vi "feedforward_estimation.vi"(2 "Parameters":T1={"Stimulus"={"Type"=enum."Off", "Phase"=0.0, "Amplitude"=[], "Injection point"=enum."Total pose", "Closed loop"=FALSE, "Offset"=[], "Tip -> world"=FALSE, "Frequency"=0.0, "Length"=0.0}, "Goal Filter A"={"Speedup max"=0.0, "Speedup thresh"=0.0, "Speedup nonlin"=0.0, "Filters"=[]}, "Mode controls"={"Hold"=FALSE, "Cancellation"=FALSE, "Goal filter"=FALSE, "Trigger"=FALSE}, "Manipulator type"=enum."Current piezo", "Manipulator calibration"={"Tool offsets"=[], "Tip light calibration"=[], "Handle light calibration"=[], "Base pivots"=[], "Output pivots"=[], "Length center"=0.0, "Workspace height"=[], "Workspace diameter"=[0.0, 0.0, 36200.0], "Linearization"=[[0.0, 0.0, 36200.0]], "Stack travel"=400.0, "Saturation pos"=375.0, "Inverse filters"=[]}, "Network"={"Remote Host"="", "Send Status"=FALSE, "Send Port"=0, "Recv Commands"=FALSE, "Recv Port"=0}, "Goal Filter B"={"Speedup max"=0.0, "Speedup thresh"=0.0, "Speedup nonlin"=0.0, "Filters"=[]}, "Cancellation"={"KP"={"XY"=0.0, "Rxy"=0.0, "Z"=0.0, "Rz"=0.0}, "KI"=0.0, "KD"={"XY"=0.0, "Rxy"=0.0, "Z"=0.0, "Rz"=0.0}, "Max vel"=0.0, "Max acc"=0.0, "Int error limit"=0.0, "RCM gain"=0.0, "Bypass"=FALSE, "Degraded gain"=0.0}, "Transition time"=0.0, "Estimation"={"Link"={"Measure noise"=[], "Process noise"=[], "Alt process noise"=[], "Alt turnoff cycles"=20, "Innovation limit"=[], "Residue threshold"=0.0, "Enable"=FALSE}, "Handle"={"Measure noise"=[], "Process noise"=[], "State limits"=[], "Innovation limit"=[], "Prediction Lookahead"=0.0, "Enable"=FALSE}}} {"Transition time" format="%_3f"; "Cancellation"."Degraded gain" min=0 max=1 step=0.1 format="%#_3p"; "Cancellation"."RCM gain" min=0 max=1 step=0.1 format="%#_3p"; "Cancellation"."KD"."Rz" min=0 max=1 step=0.1 format="%#_3p"; "Cancellation"."KD"."Rxy" min=0 max=1 step=0.1 format="%#_3p"; "Cancellation"."KD"."Z" min=0 max=1 step=0.1 format="%#_3p"; "Cancellation"."KD"."XY" min=0 max=1 step=0.1 format="%#_3p"; "Cancellation"."KI" min=0 max=1 step=0.01 format="%#_3p"; "Cancellation"."KP"."Rz" min=0 max=1 step=0.1 format="%#_3p"; "Cancellation"."KP"."Rxy" min=0 max=1 step=0.1 format="%#_3p"; "Cancellation"."KP"."Z" min=0 max=1 step=0.1 format="%#_3p"; "Cancellation"."KP"."XY" min=0 max=1 step=0.1 format="%#_3p"; "Cancellation"."Max acc" format="%#_3p"; "Goal Filter B"."Filters"."V limit range" format="%_3p"; "Goal Filter B"."Filters"."V limit" format="%_3p"; "Goal Filter B"."Filters"."Upper Q" format="%_3f"; "Goal Filter B"."Filters"."Upper Fc" format="%_3p"; "Goal Filter B"."Filters"."Lower Q" format="%_3f"; "Goal Filter B"."Filters"."Scale factor" format="%_3f"; "Goal Filter B"."Filters"."Lower Fc" format="%_3p"; "Goal Filter B"."Speedup nonlin" format="%_3p"; "Goal Filter B"."Speedup thresh" format="%_3p"; "Goal Filter B"."Speedup max" format="%_3p"; "Manipulator calibration"."Saturation pos" format="%#.1f"; "Manipulator calibration"."Stack travel" format="%#.1f"; "Manipulator calibration"."Output pivots" format="%#_6f"; "Manipulator calibration"."Base pivots" format="%#_6f"; "Manipulator calibration"."Handle light calibration" format="%#.1f"; "Manipulator calibration"."Tip light calibration" format="%#.1f"; "Goal Filter A"."Filters"."V limit range" format="%_3p"; "Goal Filter A"."Filters"."V limit" format="%_3p"; "Goal Filter A"."Filters"."Upper Q" format="%_3f"; "Goal Filter A"."Filters"."Upper Fc" format="%_3p"; "Goal Filter A"."Filters"."Lower Q" format="%_3f"; "Goal Filter A"."Filters"."Scale factor" format="%_3f"; "Goal Filter A"."Filters"."Lower Fc" format="%_3p"; "Goal Filter A"."Speedup nonlin" format="%_3p"; "Goal Filter A"."Speedup thresh" format="%_3p"; "Goal Filter A"."Speedup max" format="%_3p"; "Stimulus"."Length" min=0.0 max=100.0 step=100.0 format="%#_4p"; "Stimulus"."Frequency" min=0.0 step=100.0 format="%#_4g"; "Stimulus"."Offset" format="%#_3p"; "Stimulus"."Amplitude" format="%#_3p"; "Stimulus"."Phase" min=-180.0 max=360.0 step=100.0 format="%#.2f"}, 3 "Handle Velocity":dbl[](array[numeric]), 4 "Handle Acceleration":dbl[](array[numeric])) -> (5 "Prediction":dbl[](array[numeric]))   [LabVIEW 2013]
uses:
  <vilib>/Analysis/NI_AALBase.lvlib
  <vilib>/Analysis/baseanly.llb/A x Vector.vi
  testing/injection_point.ctl
  testing/stimulus.ctl
  testing/mode_conrols.ctl
  asap/labview/testing/probe_calibration.ctl
  testing/manipulator_cal.ctl
  host/network_params.ctl
  testing/Micron params.ctl
  goal_loop_parms.ctl
  cancellation/decoupled_gain.ctl
  cancellation/sq_control_params.ctl
  cancellation/estimation_controls.ctl
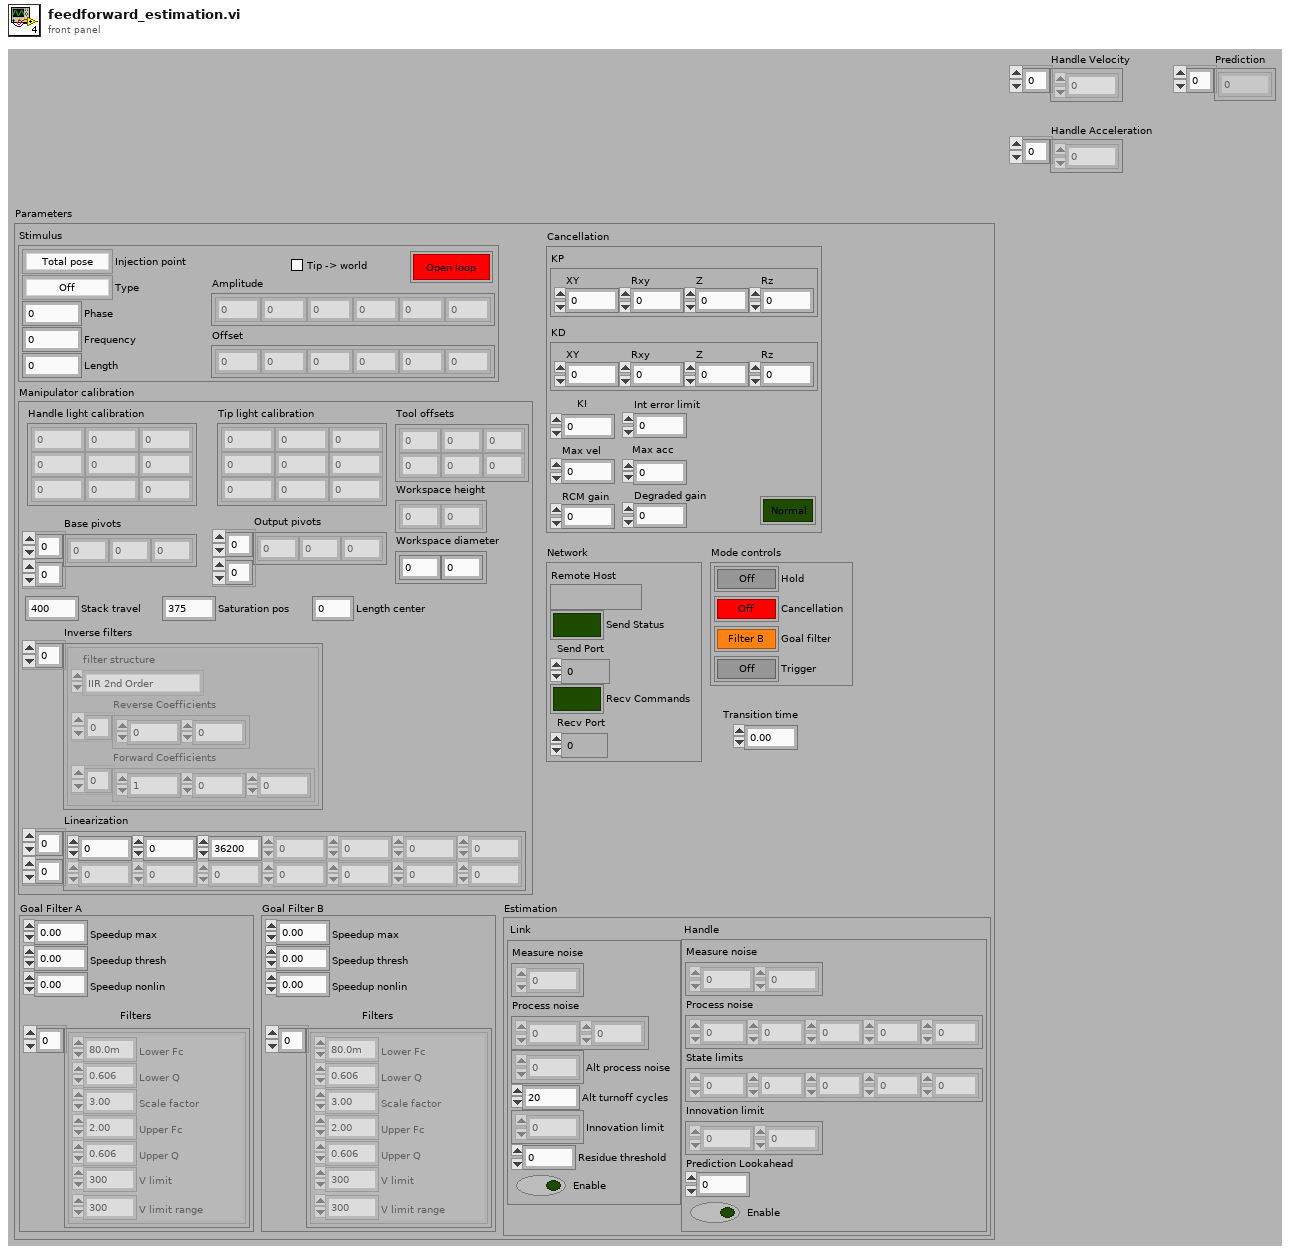
[diagram p1: front panel]
types:
  T1 = typedef "Micron params.ctl" = cluster{"Stimulus":T2, "Goal Filter A":T4, "Mode controls":T5, "Manipulator type":enum16{"Current piezo", "Voltage piezo"}, "Manipulator calibration":T6, "Network":T8, "Goal Filter B":T4, "Cancellation":T9, "Transition time":sgl, "Estimation":T11}
  T2 = typedef "stimulus.ctl" = cluster{"Type":enum16{"Off", "Step", "Sine", "Triangle", "Arbitrary"}, "Phase":dbl, "Amplitude":sgl[], "Injection point":T3, "Closed loop":bool, "Offset":sgl[], "Tip -> world":bool, "Frequency":dbl, "Length":dbl}
  T3 = typedef "injection_point.ctl" = enum16{"Total pose", "V limiter", "Goal ", "Link position", "KF link position", "Inverse kin", "Link goal", "Link error", "Controller", "Output", "Drive", "Light"}
  T4 = typedef "goal_loop_parms.ctl" = cluster{"Speedup max":sgl, "Speedup thresh":sgl, "Speedup nonlin":sgl, "Filters":cluster{"Lower Fc":sgl, "Lower Q":sgl, "Scale factor":sgl, "Upper Fc":sgl, "Upper Q":sgl, "V limit":sgl, "V limit range":sgl}[]}
  T5 = typedef "mode_conrols.ctl" = cluster{"Hold":bool, "Cancellation":bool, "Goal filter":bool, "Trigger":bool}
  T6 = typedef "manipulator_cal.ctl" = cluster{"Tool offsets":sgl[][], "Tip light calibration":T7, "Handle light calibration":T7, "Base pivots":sgl[][], "Output pivots":sgl[][], "Length center":sgl, "Workspace height":sgl[], "Workspace diameter":sgl[], "Linearization":sgl[][], "Stack travel":sgl, "Saturation pos":sgl, "Inverse filters":cluster{"filter structure":enum32{"IIR 2nd Order", "IIR 4th Order"}, "Reverse Coefficients":dbl[], "Forward Coefficients":dbl[]}[]}
  T7 = typedef "probe_calibration.ctl" = sgl[][]
  T8 = typedef "network_params.ctl" = cluster{"Remote Host":string, "Send Status":bool, "Send Port":u16, "Recv Commands":bool, "Recv Port":u16}
  T9 = typedef "sq_control_params.ctl" = cluster{"KP":T10, "KI":sgl, "KD":T10, "Max vel":sgl, "Max acc":sgl, "Int error limit":sgl, "RCM gain":sgl, "Bypass":bool, "Degraded gain":sgl}
  T10 = typedef "decoupled_gain.ctl" = cluster{"XY":sgl, "Rxy":sgl, "Z":sgl, "Rz":sgl}
  T11 = typedef "estimation_controls.ctl" = cluster{"Link":cluster{"Measure noise":dbl[], "Process noise":dbl[], "Alt process noise":dbl[], "Alt turnoff cycles":i32, "Innovation limit":dbl[], "Residue threshold":dbl, "Enable":bool}, "Handle":cluster{"Measure noise":dbl[], "Process noise":dbl[], "State limits":dbl[], "Innovation limit":dbl[], "Prediction Lookahead":sgl, "Enable":bool}}
  T12 = typedef "NI_Matrix.lvlib/RealMatrix.ctl" = dbl[][]
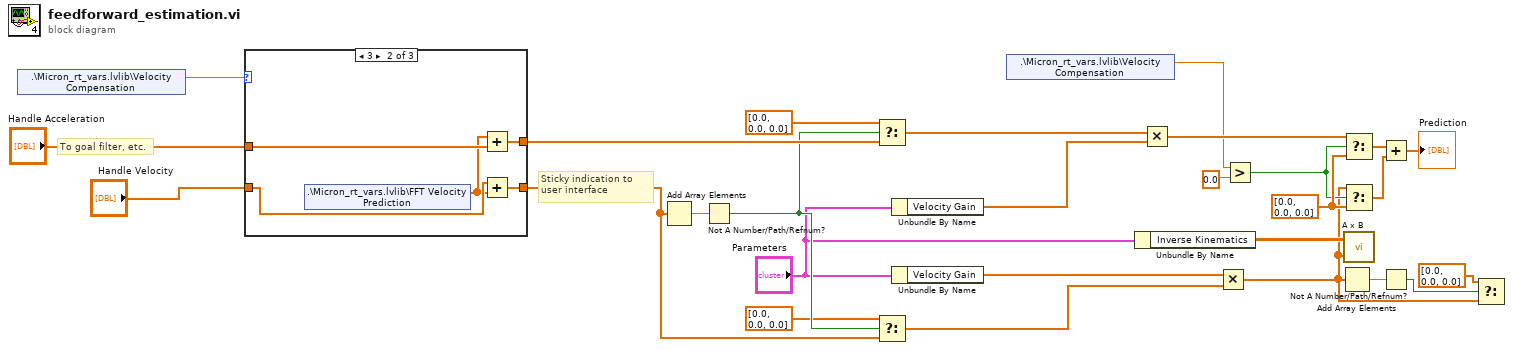
[diagram p0: block diagram]
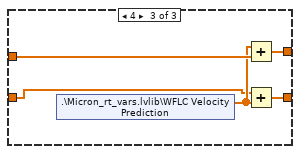
[diagram p3: hidden frame]
diagram:
  w17 = dbl[] [0.0, 0.0, 0.0] ("s? t:f")
  # "Sticky indication to user interface"
  # "To goal filter, etc."
  n1 = shared-variable ".\\Micron_rt_vars.lvlib\\Velocity Compensation"() -> (w23:sgl)  [unwired: 1 in, 1 out]
  n2 = case shown="3" w23 {
    tunnel: "Handle Acceleration" -> [w29 w34 w39]
    tunnel: [w29 w33 w38] -> w25
    tunnel: "Handle Velocity" -> [w28 w32 w36]
    tunnel: [w28 w30 w35] -> w27
    frame 0, Default {
    }
    frame 3 {
      n3 = shared-variable ".\\Micron_rt_vars.lvlib\\FFT Velocity Prediction"() -> (w31:sgl[])  [unwired: 1 in, 1 out]
      n4 = Add(x=w31, y=w34) -> (x+y=w33:dbl[])
      n5 = Add(x=w32, y=w31) -> (x+y=w30:dbl[])
    }
    frame 4 {
      n6 = shared-variable ".\\Micron_rt_vars.lvlib\\WFLC Velocity Prediction"() -> (w37:sgl[])  [unwired: 1 in, 1 out]
      n7 = Add(x=w37, y=w39) -> (x+y=w38:dbl[])
      n8 = Add(x=w36, y=w37) -> (x+y=w35:dbl[])
    }
  }
  n9 = Add Array Elements(numeric array=w27) -> (sum=w6:dbl)
  n10 = Not A Number/Path/Refnum?(number/path/refnum=w6) -> (NaN/Path/Refnum?=w14:bool)
  n11 = Select(t=dbl[] [0.0, 0.0, 0.0] ("s? t:f"), s=w14, f=w25) -> (s? t:f=w15:dbl[])
  n12 = Select(t=dbl[] [0.0, 0.0, 0.0] ("s? t:f"), s=w14, f=w27) -> (s? t:f=w7:dbl[])
  n13 = Unbundle By Name("Parameters") -> ("Velocity Gain"=w1:dbl[])
  n14 = Unbundle By Name("Parameters") -> ("Velocity Gain"=w3:dbl[])
  n15 = shared-variable ".\\Micron_rt_vars.lvlib\\Velocity Compensation"() -> (w9:sgl)  [unwired: 1 in, 1 out]
  n16 = Unbundle By Name("Parameters") -> ("Inverse Kinematics"=w20:T12)
  n17 = Multiply(x=w15, y=w1) -> (x*y=w18:dbl[])
  n18 = Multiply(x=w3, y=w7) -> (x*y=w11:dbl[])
  n19 = Greater?(x=w9, y=sgl 0.0 ("length")) -> (0:w16:bool)
  n20 = Add Array Elements(numeric array=w11) -> (sum=w4:dbl)
  n21 = Select(t=w18, s=w16, f=w17) -> (s? t:f=w19:dbl[])
  n22 = Select(t=w11, s=w16, f=w17) -> (s? t:f=w12:dbl[])
  n23 = call-poly <vilib>:"A x B.vi"("Vector"=w11, "A"=w20) -> ()  [unwired: 2 out]
  n24 = Add(x=w19, y=w12) -> (x+y=→"Prediction":dbl[])
  n25 = Not A Number/Path/Refnum?(number/path/refnum=w4) -> (NaN/Path/Refnum?=w5:bool)
  n26 = Select(t=dbl[] [0.0, 0.0, 0.0] ("s? t:f"), s=w5, f=w11) -> ()  [unwired: 1 out]
